vi "Skaluj_przebieg_Kursor.vi"(6 "Przebiegi Monit":T1, 7 "Pomiarowe OK? in":bool, 8 "error in (no error)":errorcluster, 11 "WaveformGraph in":refnum<vi>) -> (0 "error out":errorcluster, 2 "Plot.YScaleIdx":u32, 3 "Pomiarowe OK? out":bool)   [LabVIEW 2013]
doc: "Sprawdza czy dwa przebiegi pomiarowe są na tej samej skali,\nwtedy przerzuca przegieg Kursor na tą samą skalę"
uses:
  dwa_przebiegi_.ctl
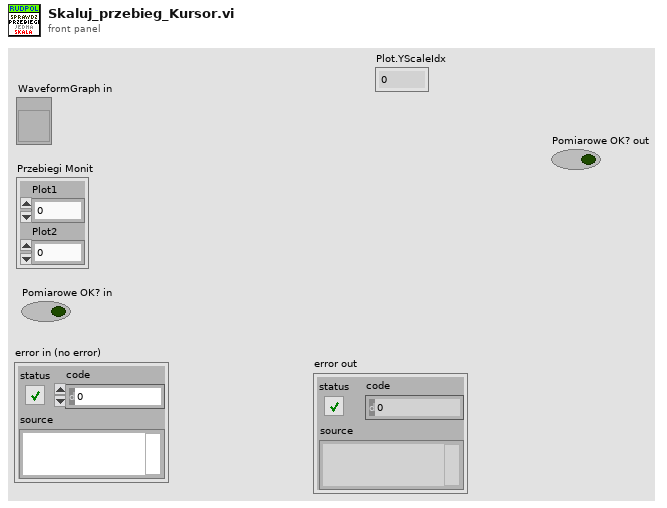
[diagram p1: front panel]
types:
  T1 = typedef "dwa_przebiegi_.ctl" = cluster{"Plot1":i32, "Plot2":i32}
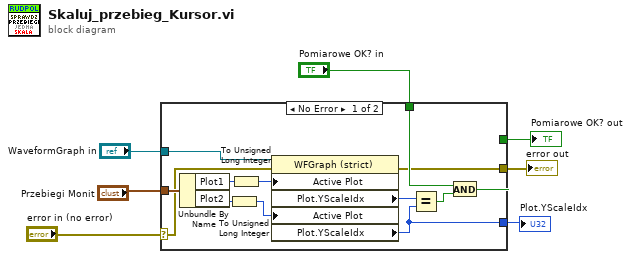
[diagram p0: block diagram]
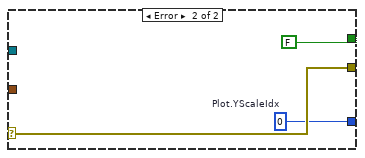
[diagram p2: hidden frame]
diagram:
  n1 = case shown="No Error" "error in (no error)" {
    selector: "error in (no error)" -> [w11 w23]
    tunnel: "WaveformGraph in" -> [w17 _]
    tunnel: "Pomiarowe OK? in" -> [w16 _]
    tunnel: "Przebiegi Monit" -> [w12 _]
    tunnel: [w10 w23] -> w3
    tunnel: [w9 FALSE] -> w2
    tunnel: [w8 w21] -> w1
    frame No Error {
      n2 = Unbundle By Name(w12) -> ("Plot1"=w13:i32, "Plot2"=w14:i32)
      n3 = To Unsigned Long Integer(number=w14) -> (unsigned 32bit integer=w20:u32)
      n4 = To Unsigned Long Integer(number=w13) -> (unsigned 32bit integer=w18:u32)
      n5 = property class="WFGraph (strict)"(reference=w17, error in=w11, "Active Plot"=w18, "Active Plot"=w20) -> (error out=w10:errorcluster, "Plot.YScaleIdx"=w19:u32, "Plot.YScaleIdx"=w8:u32)  [unwired: 1 out]
      n6 = Equal?(x=w19, y=w8) -> (x = y?=w15:bool)
      n7 = And(x=w16, y=w15) -> (x .and. y?=w9:bool)
    }
    frame Error {
      w21 = u32 0  # Plot.YScaleIdx
    }
  }
  "error out" <- w3
  "Pomiarowe OK? out" <- w2
  "Plot.YScaleIdx" <- w1
